vi "Write sequence state.vi"(8 "error in (no error)":errorcluster, 10 "sequence state":T1, 11 "Change Sequence State MSG in":refnum<class "Change Sequence State MSG.lvclass">) -> (0 "error out":errorcluster, 3 "Change Sequence State MSG out":refnum<class "Change Sequence State MSG.lvclass">)   [LabVIEW 2017, in "Controller.lvlib" / "Change Sequence State MSG.lvclass"]
uses:
  Change Sequence State MSG.lvclass
  Sequencer/sequenceState.ctl
  Change Sequence State MSG.lvclass/Change Sequence State MSG.ctl
  Controller.lvlib
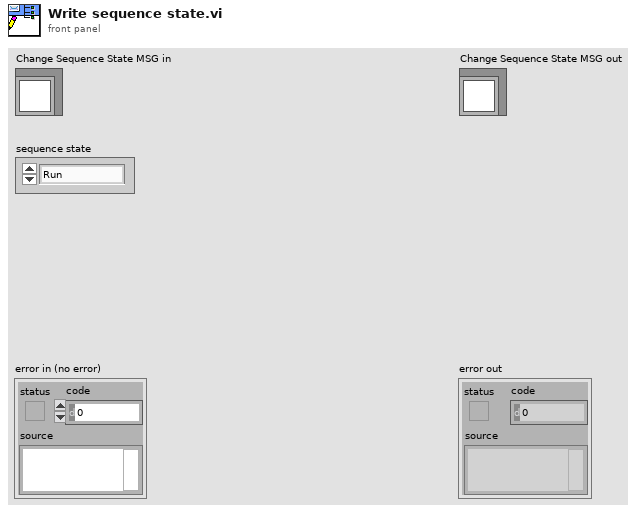
[diagram p1: front panel]
types:
  T1 = typedef "Controller.lvlib/sequenceState.ctl" = enum16{"Run", "Pause", "Reset", "Reload", "Stop"}
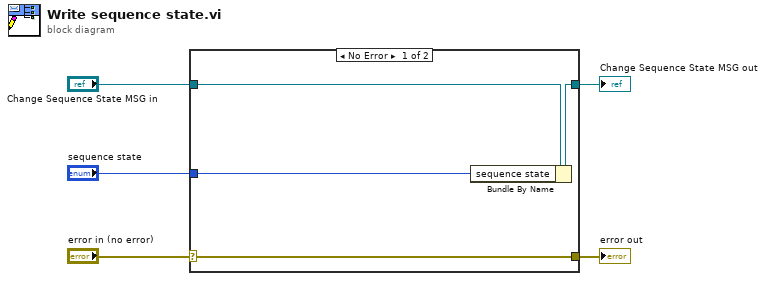
[diagram p0: block diagram]
diagram:
  n1 = case shown="No Error" "error in (no error)" {
    selector: "error in (no error)" -> [w9 w10]
    tunnel: [w9 w10] -> w4
    tunnel: [w7 w11] -> w2
    tunnel: "Change Sequence State MSG in" -> [w8 w11]
    tunnel: "sequence state" -> [w6 _]
    frame No Error {
      n2 = Bundle By Name(cluster=w8, "sequence state"=w6) -> (w7:refnum<class "Change Sequence State MSG.lvclass">)
    }
    frame Error {
    }
  }
  "error out" <- w4
  "Change Sequence State MSG out" <- w2
